vi "SOS.vi"(8 "channel":T3, 9 "channel for IA State":T2, 10 "channel 2":T1, 11 "channel in":T2) -> (0 "channel  out 3":T2, 1 "channel  out 4":T1, 2 "channel  out 2":T3, 3 "channel  out":T2)   [LabVIEW 2016]
uses:
  <extravilib>/ChannelInstances/Lossy Stream-t'AI Input.ctl'/)Channel.ctl
  Core/AI Input.ctl
  Core/AI Robot.ctl
  Intel/Functions Enum.ctl
  Intel/AttackerStates.ctl
  Core/AI Ball.ctl
  Core/Field Size.ctl
  Core/AI Judge.ctl
  Intel/Command Enum.ctl
  Util/Events/Events.ctl
  DrawTargets.ctl
  <extravilib>/ChannelInstances/Lossy Stream-t'SSL Field State.ctl'/)Channel.ctl
  SSL/SSL Field State.ctl
  SSL Detection Frame.ctl
  SSL Detection Robot.ctl
  <vilib>/Analysis/Matrix/Datatypes/RealMatrix.ctl
  SSL Detection Ball.ctl
  <extravilib>/ChannelInstances/Lossy Stream-a[.](i32)/)Channel.ctl
  <vilib>/Analysis/_algsub.llb/Real Vector Norm.vi
  <extravilib>/ChannelInstances/Lossy Stream-a[.](i32)/Read With Abort.vi
  <extravilib>/ChannelInstances/Lossy Stream-a[.](i32)/Write With Abort.vi
  <extravilib>/ChannelInstances/Lossy Stream-t'AI Input.ctl'/Read With Abort.vi
  <extravilib>/ChannelInstances/Lossy Stream-t'AI Input.ctl'/Write With Abort.vi
  <extravilib>/ChannelInstances/Lossy Stream-t'SSL Field State.ctl'/Read With Abort.vi
  <extravilib>/ChannelInstances/Lossy Stream-t'SSL Field State.ctl'/Write With Abort.vi
  <extravilib>/ChannelInstances/Lossy Stream-a[.](i32)/Endpoint.vi
  <extravilib>/ChannelInstances/Lossy Stream-t'AI Input.ctl'/Endpoint.vi
  <extravilib>/ChannelInstances/Lossy Stream-t'SSL Field State.ctl'/Endpoint.vi
  <extravilib>/ChannelInstances/Lossy Stream-t'AI Input.ctl'/)Channel.vi
  <resource>/ChannelSupport/_ChannelSupport/WaitIfNeeded.vi
  <extravilib>/ChannelInstances/Lossy Stream-t'SSL Field State.ctl'/)Channel.vi
  <extravilib>/ChannelInstances/Lossy Stream-a[.](i32)/)Channel.vi
  <extravilib>/ChannelInstances/Lossy Stream-a[.](i32)/Instantiate.vi
  <extravilib>/ChannelInstances/Lossy Stream-t'AI Input.ctl'/Instantiate.vi
  <extravilib>/ChannelInstances/Lossy Stream-t'SSL Field State.ctl'/Instantiate.vi
  <extravilib>/ChannelInstances/Lossy Stream-t'AI Input.ctl'.lvlib
  <vilib>/Analysis/NI_AALPro.lvlib
  <extravilib>/ChannelInstances/Lossy Stream-t'SSL Field State.ctl'.lvlib
  <extravilib>/ChannelInstances/Lossy Stream-a[.](i32).lvlib
  <vilib>/Analysis/Matrix/NI_Matrix.lvlib
panel:
  in  "Draw Targets?":T4={"Attacker"=TRUE, "Striker"=TRUE, "Goalie"=TRUE, "Defender"=TRUE, "kick"=TRUE, "Est Ball"=TRUE, "Est Robot"=FALSE}
  in  "ID robô inimigo":dbl
  in  "ID robô":dbl
  in  "Velocidade bola":bool
  in  "Velocidade robô inimigo":bool
  in  "Velocidade robô":bool
  out "Vel_Enemy_Robots":dbl(graph)
  out "Vel_Robots":dbl(graph)
  out "Vel_Ball":dbl(graph)
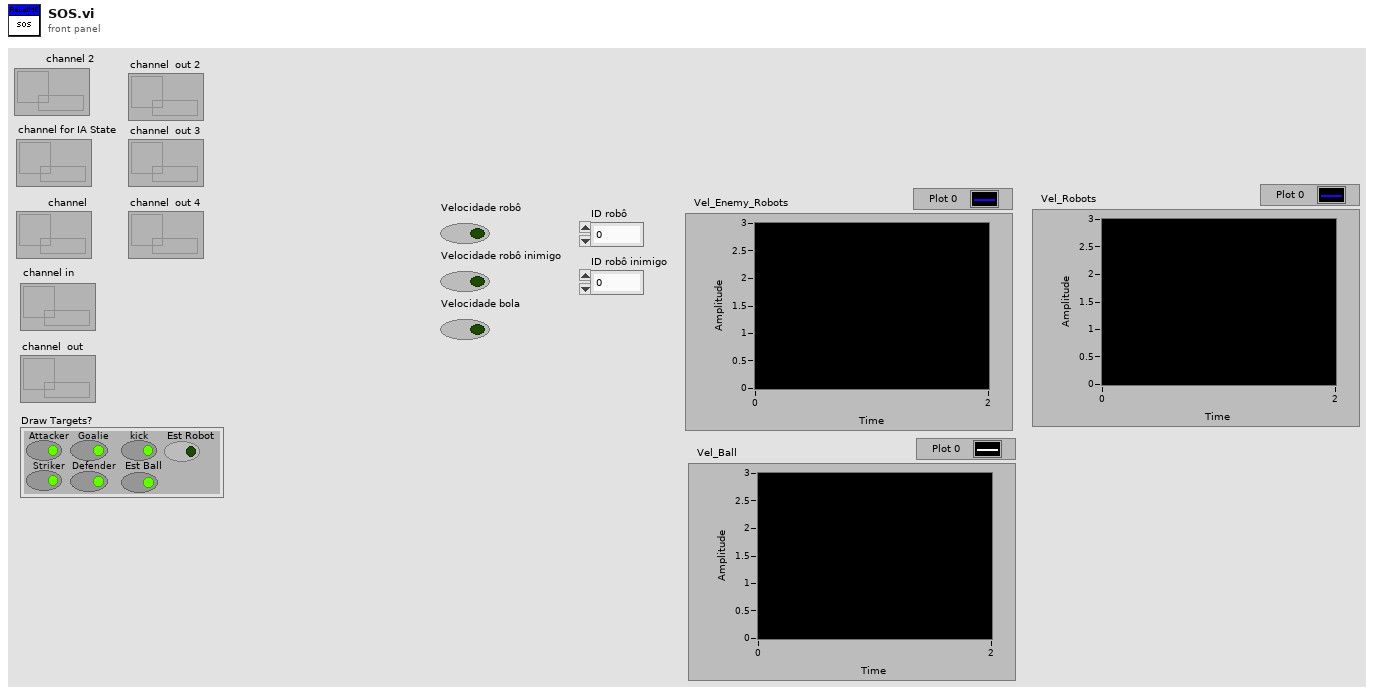
[diagram p1: front panel]
types:
  T1 = typedef "Lossy Stream-a[.](i32).lvlib/)Channel.ctl" = refnum<queue>
  T2 = typedef "Lossy Stream-t'AI Input.ctl'.lvlib/)Channel.ctl" = refnum<queue>
  T3 = typedef "Lossy Stream-t'SSL Field State.ctl'.lvlib/)Channel.ctl" = refnum<queue>
  T4 = typedef "DrawTargets.ctl" = cluster{"Attacker":bool, "Striker":bool, "Goalie":bool, "Defender":bool, "kick":bool, "Est Ball":bool, "Est Robot":bool}
  T5 = typedef "AI Input.ctl" = cluster{"our_robots":T6[], "enemy_robots":T6[], "balls":T9[], "geometry":T10, "IA Judge":T11, "Received Timestamp":timestamp, "Events":T13}
  T6 = typedef "AI Robot.ctl" = cluster{"id":u32, "function":T7, "x":dbl, "y":dbl, "orientation":dbl, "v_tangent":dbl, "v_normal":dbl, "v_ang":dbl, "kick_x":dbl, "kick_z":dbl, "dribble":bool, "Timestamp":timestamp, "dest_x":dbl, "dest_y":dbl, "dest_orientation":dbl, "estimatives":cluster{"est_v_tangent":dbl, "est_v_normal":dbl, "est_vx":dbl, "est_vy":dbl, "Pos Robot Est":dbl[]}, "dest_x_kick":dbl, "dest_y_kick":dbl, "Gap Coord":dbl[], "States":T8}
  T7 = typedef "Functions Enum.ctl" = enum16{"Attacker", "Goalie", "Defender", "Striker", "Goto 0", "Dummy", "Kicker", "ZigZag"}
  T8 = typedef "AttackerStates.ctl" = enum16{"Pass", "GoToTangent", "BallGetting", "GoToKick", ""}
  T9 = typedef "AI Ball.ctl" = cluster{"x":dbl, "y":dbl, "timestamp":timestamp, "Vel_x":dbl, "Vel_y":dbl, "Pos Bola Est":dbl[]}
  T10 = typedef "Field Size.ctl" = cluster{"line_width":u32, "field_length":u32, "field_width":u32, "boundary_width":u32, "referee_width":u32, "goal_width":u32, "goal_depth":u32, "goal_wall_width":u32, "center_circle_radius":u32, "defense_radius":u32, "defense_stretch":u32, "free_kick_from_defense_dist":u32, "penalty_spot_from_field_line_dist":u32, "penalty_line_from_spot_dist":u32}
  T11 = typedef "AI Judge.ctl" = cluster{"stage":string, "command":string, "our_goalie_id":dbl, "enemy_goalie_id":dbl, "command enum":T12, "Time":enum16{"Azul", "Amarelo"}}
  T12 = typedef "Command Enum.ctl" = enum16{"Halt", "Stop", "Force Start", "PKA Normal Start", "Prepare Kickoff Ally", "PKE Normal Start", "Prepare Kickoff Enemy", "Prepare Penalty Ally", "PPA Normal Start", "Prepare Penalty Enemy", "PPE Normal Start", "Direct Free Enemy", "Direct Free Ally", "Indirect Free Enemy", "Indirect Free Ally", "Timeout Enemy", "Timeout Ally", "Goal Enemy", "Goal Ally", "Ball Placement Enemy", "Ball Placement Ally", "Normal Half Time", "Extra Time Break", "Extra Half Time", "None", "Post Game"}
  T13 = typedef "Events.ctl" = cluster{"Touch":bool, "Ball out":bool, "id touch":dbl, "Ball out of \nVision":bool, "Ball inside \nGoalie area":bool, "Robot not responding":bool, "Robots responding status":dbl[], "Enemy Ball \nPossession":bool, "Pass State":bool, "id end of pass":dbl, "Kick":bool, "Id ini Possession":dbl, "Ball Possesion":bool, "Id Possesion":dbl}
  T14 = typedef "SSL Field State.ctl" = cluster{"Detection Frame Out":T15, "Field Size Out":cluster{"line_width":u32, "field_length":u32, "field_width":u32, "boundary_width":u32, "referee_width":u32, "goal_width":u32, "goal_depth":u32, "goal_wall_width":u32, "center_circle_radius":u32, "defense_radius":u32, "defense_stretch":u32, "free_kick_from_defense_dist":u32, "penalty_spot_from_field_line_dist":u32, "penalty_line_from_spot_dist":u32}, "Received Time Stamp":timestamp}
  T15 = typedef "SSL Detection Frame.ctl" = cluster{"frame_number":u32, "t_capture":dbl, "t_sent":dbl, "camera_id":u32, "robots_yellow":T16[], "robots_blue":T16[], "balls":T18[], "Valid":bool, "Time Stamp":timestamp}
  T16 = typedef "SSL Detection Robot.ctl" = cluster{"x":sgl, "robot_id":u32, "confidence":sgl, "y":sgl, "orientation":sgl, "pixel_x":sgl, "pixel_y":sgl, "height":sgl, "Valid":bool, "Time Stamp":timestamp, "x_k|k":T17, "Pk|k":T17, "Previous Time Stamp":timestamp, "R":T17}
  T17 = typedef "NI_Matrix.lvlib/RealMatrix.ctl" = dbl[][]
  T18 = typedef "SSL Detection Ball.ctl" = cluster{"x":sgl, "area":u32, "confidence":sgl, "y":sgl, "z":sgl, "pixel_x":sgl, "pixel_y":sgl, "Valid":bool, "Time Stamp":timestamp, "x_k|k":T17, "Pk|k":T17, "Id":u32, "Previous Time Stamp":timestamp, "R":T17}
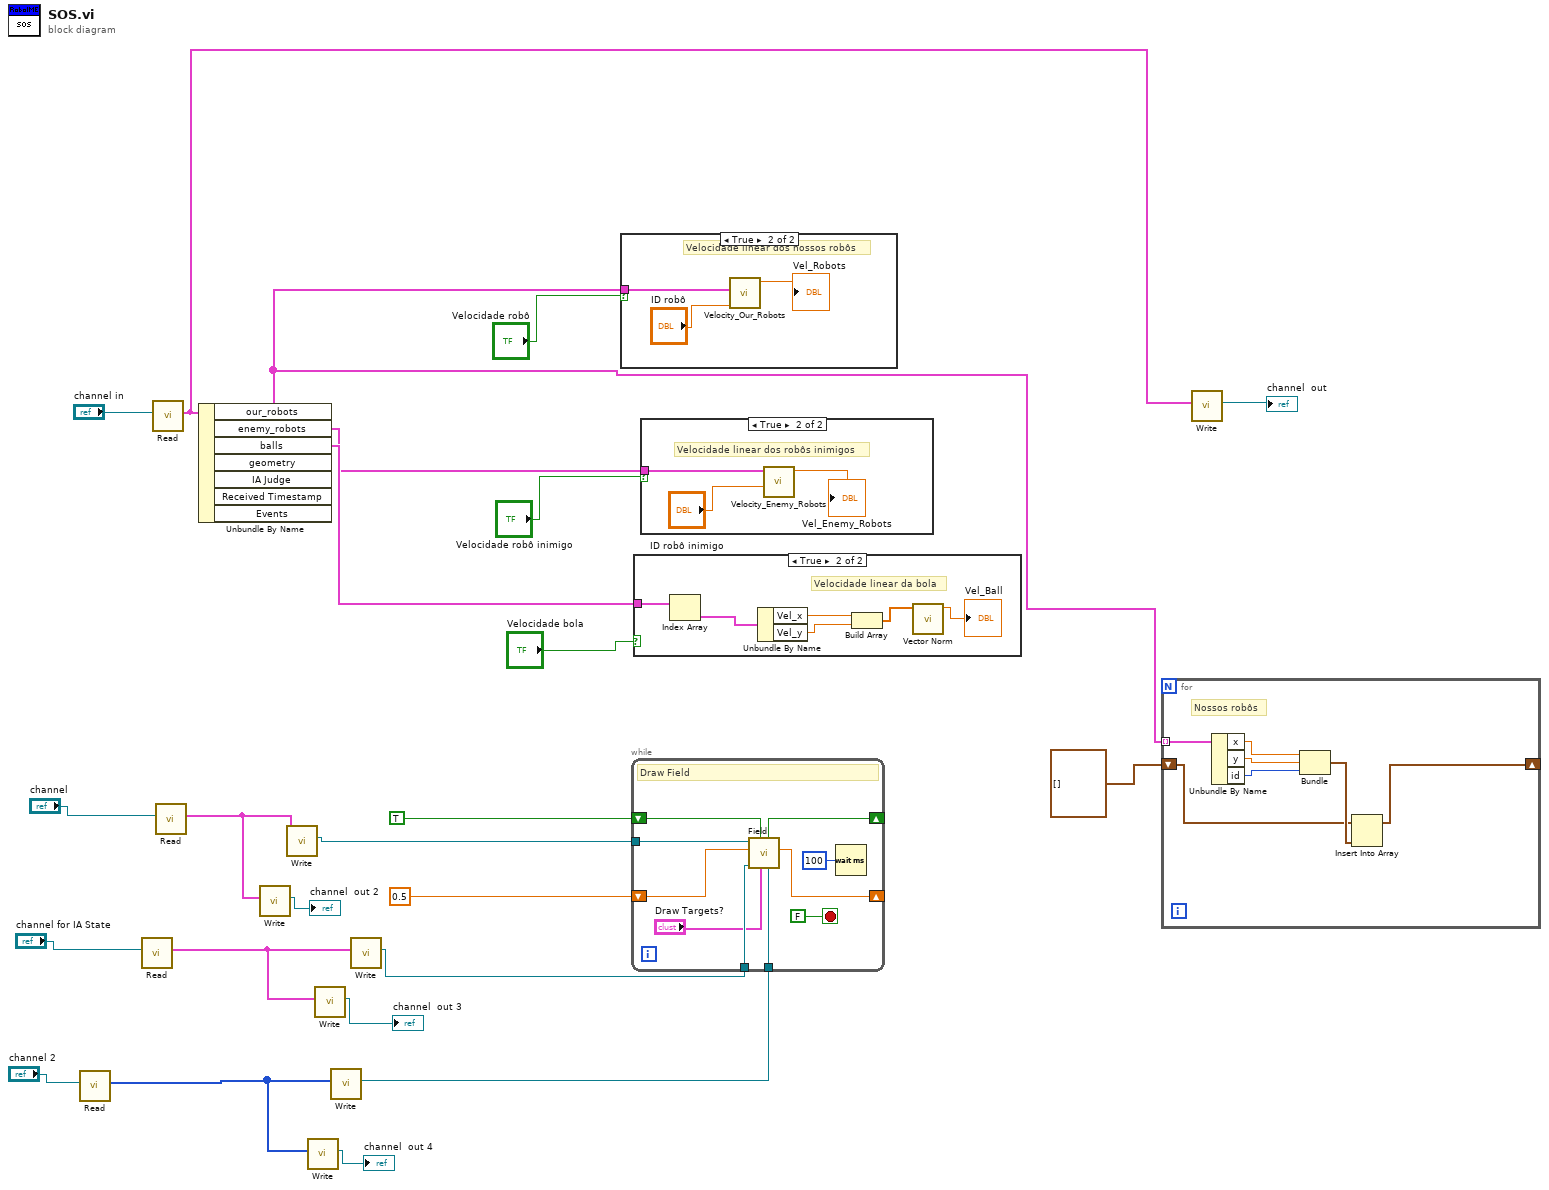
[diagram p0: block diagram]
diagram:
  n1 = call <extravilib>:"Read.vi"("channel"="channel 2") -> ("element"=w6:i32[])  [unwired: 5 in, 5 out]
  n2 = call <extravilib>:"Read.vi"("channel"="channel for IA State") -> ("element"=w7:T5)  [unwired: 5 in, 5 out]
  n3 = call <extravilib>:"Read.vi"("channel"="channel in") -> ("element"=w22:T5)  [unwired: 5 in, 5 out]
  n4 = call <extravilib>:"Read.vi"("channel"="channel") -> ("element"=w13:T14)  [unwired: 5 in, 5 out]
  n5 = Unbundle By Name(w22) -> ("our_robots"=w2:T6[], "enemy_robots"=w20:T6[], "balls"=w23:T9[])  [unwired: 4 out]
  n6 = call <extravilib>:"Write.vi"("element"=w13) -> ("channel"=→"channel  out 2":T3)  [unwired: 8 in, 2 out]
  n7 = call <extravilib>:"Write.vi"("element"=w13) -> ("channel"=w12:T3)  [unwired: 8 in, 2 out]
  n8 = call <extravilib>:"Write.vi"("element"=w6) -> ("channel"=→"channel  out 4":T1)  [unwired: 8 in, 2 out]
  n9 = call <extravilib>:"Write.vi"("element"=w7) -> ("channel"=→"channel  out 3":T2)  [unwired: 8 in, 2 out]
  n10 = call <extravilib>:"Write.vi"("element"=w6) -> ("channel"=w8:T1)  [unwired: 8 in, 2 out]
  n11 = call <extravilib>:"Write.vi"("element"=w7) -> ("channel"=w9:T2)  [unwired: 8 in, 2 out]
  n12 = case shown="True" "Velocidade robô" {
    tunnel: w2 -> [_ w27]
    frame False {
    }
    frame True {
      # "Velocidade linear dos nossos robôs"
      n13 = call "Velocity_Our_Robots.vi"("Robot_ID"="ID robô", "our_robots"=w27) -> ("Vel_Robots"=→"Vel_Robots":dbl)  [unwired: 9 in]
    }
  }
  n14 = while {
    shift-right: [w36] -> _
    shift-left: 0.5 ("New Scale") -> [w30]
    shift-right: [w35] -> _
    shift-left: TRUE ("AutoScale Out") -> [w34]
    tunnel: w9 -> [w32]
    tunnel: w12 -> [w31]
    tunnel: w8 -> [w29]
    stop <- FALSE stop-if-true
    # "Draw Field"
    n15 = call "Field.vi"("channel 2"=w29, "Draw Targets?"="Draw Targets?", "AutoScale"=w34, "channel for IA State"=w32, "Scale mm/pixel"=w30, "channel"=w31) -> ("Scale Out"=w36:dbl, "AutoScale Out"=w35:bool)  [unwired: 3 in, 1 out]
    n16 = Wait (ms)(milliseconds to wait=u32 100) -> ()  [unwired: 1 out]
  }
  n17 = case shown="True" "Velocidade bola" {
    tunnel: w23 -> [_ w43]
    frame False {
    }
    frame True {
      # "Velocidade linear da bola"
      n18 = Index Array(array=w43) -> (element=w42:T9)  [unwired: 1 in]
      n19 = Unbundle By Name(w42) -> ("Vel_x"=w39:dbl, "Vel_y"=w38:dbl)
      n20 = Build Array(w39, w38) -> (w41:dbl[])
      n21 = call-poly <vilib>:"Vector Norm.vi"("Input Vector"=w41) -> ("norm"=→"Vel_Ball":dbl)  [unwired: 9 in, 1 out]
    }
  }
  n22 = case shown="True" "Velocidade robô inimigo" {
    tunnel: w20 -> [_ w46]
    frame False {
    }
    frame True {
      # "Velocidade linear dos robôs inimigos"
      n23 = call "Velocity_Enemy_Robots.vi"("Pick_ID"="ID robô inimigo", "enemy_robots"=w46) -> ("Vel_Enemy_Robots"=→"Vel_Enemy_Robots":dbl)  [unwired: 9 in]
    }
  }
  n24 = for {
    tunnel: w2 -> [w53] mode=indexing
    shift-right: [w48] -> _
    shift-left: cluster{"x":dbl, "y":dbl, "id":u32}[] [] -> [w47]
    # "Nossos robôs"
    n25 = Unbundle By Name(w53) -> ("x"=w52:dbl, "y"=w51:dbl, "id"=w50:u32)
    n26 = Bundle("x"=w52, "y"=w51, "id"=w50) -> (w49:cluster{"x":dbl, "y":dbl, "id":u32})  [unwired: 1 in]
    n27 = Insert Into Array(array=w47, new element=w49) -> (w48:cluster{"x":dbl, "y":dbl, "id":u32}[])  [unwired: 1 in]
  }
  n28 = call <extravilib>:"Write.vi"("element"=w22) -> ("channel"=→"channel  out":T2)  [unwired: 8 in, 2 out]
